vi "Procedure Parameters Example (B).vi"() -> ()   [LabVIEW 2011]
uses:
  C:/Program Files/Metrohm Autolab/Autolab SDK 1.10/EcoChemie.Autolab.Sdk.dll
  EcoChemie.Autolab.Sdk.dll
panel:
  in  "Stop":bool
  out "error out":errorcluster
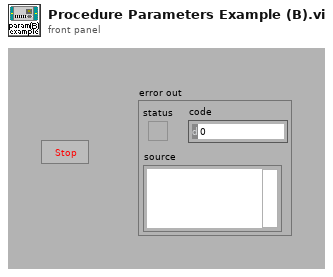
[diagram p1: front panel]
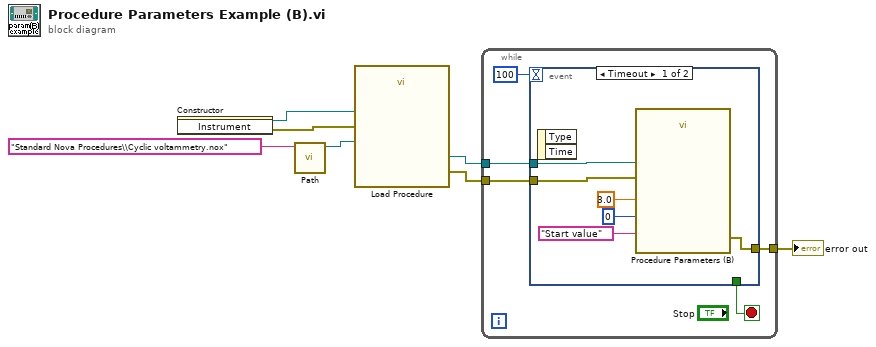
[diagram p0: block diagram]
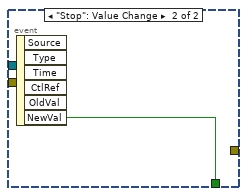
[diagram p2: hidden frame]
diagram:
  n1 = constructor class="Instrument"() -> (reference out=w4:refnum<k24>, error out=w6:errorcluster)  [unwired: 3 in, 1 out]
  n2 = call "Path.vi"("name or relative path"="Standard Nova Procedures\\Cyclic voltammetry.nox") -> ("appended path"=w5:path)  [unwired: 10 in]
  n3 = call "Load Procedure.vi"("error in (no error)"=w6, "Procedure"=w5, "Instrument"=w4) -> ("error out"=w2:errorcluster, "LoadProcedure"=w3:refnum<k24>)  [unwired: 5 in, 2 out]
  n4 = while {
    tunnel: w3 -> [w12]
    tunnel: w2 -> [w11]
    tunnel: [w10] -> w1
    stop <- w8 stop-if-true
    n5 = event shown="[0] Timeout" {
      selector: _ -> [_ _]
      dyn-events: _ -> [_ _]
      timeout: 100 ("Numeric") -> [_ _]
      tunnel: w12 -> [w15 _]
      tunnel: w11 -> [w14 _]
      tunnel: [w13 _] -> w10
      tunnel: [_ w19] -> w8
      event Timeout {
        n6 = event-data() -> ()  [unwired: 1 in, 2 out]
        n7 = call "Procedure Parameters (B).vi"("LoadProcedure"=w15, "Command Parameter"="Start value", "IntSet"=0, "DoubleSet"=3.0, "error in (no error)"=w14) -> ("error out"=w13:errorcluster)  [unwired: 10 in]
      }
      event "Stop": Value Change {
        n8 = event-data() -> ("NewVal"=w19:bool)  [unwired: 1 in, 5 out]
      }
    }
  }
  "error out" <- w1
